vi "Scratch Test.vi"() -> ()   [LabVIEW 2020, in "Vecto.lvlib" / "IP Resolver.lvclass"]
uses:
  IP Resolver.lvclass
  Bind Info.ctl
  Address Type.ctl
  IP Target.ctl
  IP Resolver.lvclass/IP Resolver.ctl
panel:
  in  "IP Target":T1
  out "error out":errorcluster
  out "IP":string
  out "Info":T2[](array[typedef])
  in  "Bindings":string[](array[string])
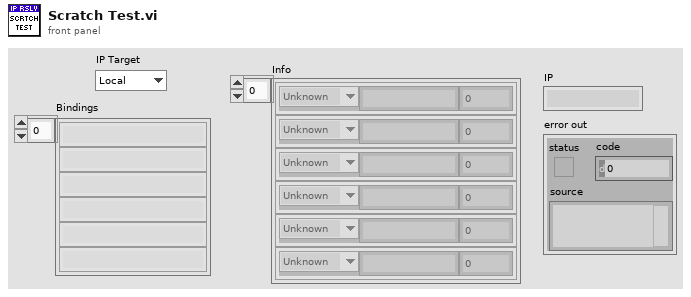
[diagram p1: front panel]
types:
  T1 = typedef "Vecto.lvlib/IP Resolver.lvclass/IP Target.ctl" = enum16{"Local", "External"}
  T2 = typedef "Vecto.lvlib/IP Resolver.lvclass/Bind Info.ctl" = cluster{"Type":T3, "Binding":string, "Subnet Bits":i32}
  T3 = typedef "Vecto.lvlib/IP Resolver.lvclass/Address Type.ctl" = enum16{"Unknown", "Specific", "Subnet", "Any"}
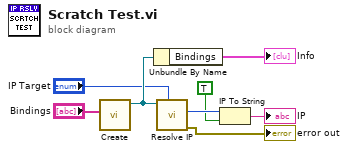
[diagram p0: block diagram]
diagram:
  n1 = call "Create.vi"("Bindings"="Bindings") -> ("IP Resolver out"=w6:refnum<class "IP Resolver.lvclass">)  [unwired: 9 in, 1 out]
  n2 = Unbundle By Name(w6) -> ("Bindings"=→"Info":T2[])
  n3 = call "Resolve IP.vi"("IP Target (Local)"="IP Target", "IP Resolver in"=w6) -> ("error out"=→"error out":errorcluster, "U32 Address"=w5:u32)  [unwired: 7 in, 1 out]
  n4 = IP To String(1:TRUE ("dot notation? (F)"), 2:w5) -> (0:→"IP":string)
